vi "Multify(CSG).vi"(1 "启用（T）":bool=TRUE, 2 "In":csg, 4 "n":csg=1.0+0.0i) -> (6 "Out":csg=1.0+0.0i format="%.2f")   [LabVIEW 2011]
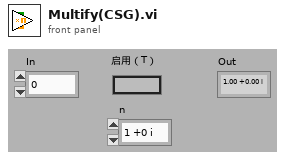
[diagram p1: front panel]
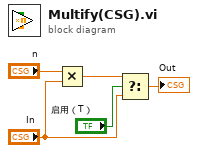
[diagram p0: block diagram]
diagram:
  n1 = Multiply(x="n", y="In") -> (x*y=w1:csg)
  n2 = Select(t=w1, s="启用（T）", f="In") -> (s? t:f=→"Out":csg)
